vi "initialise.vi"(8 "error in (no error)":errorcluster, 11 "TrajectoryAN1106117SinglePoint in":refnum<class "TrajectoryAN1106117SinglePoint.lvclass">) -> (0 "error out":errorcluster, 3 "TrajectoryAN1106117SinglePoint out":refnum<class "TrajectoryAN1106117SinglePoint.lvclass">)   [LabVIEW 2010, in "TrajectoryAN1106117SinglePoint.lvclass"]
uses:
  TrajectoryAN1106117SinglePoint.lvclass
  TrajectoryDL091126GenericVoxel/TrajectoryDL091126GenericVoxel/TrajectoryDL091126GenericVoxel.lvclass
  common/enumerations/x_y_z_enumeration.ctl
  common/enumerations/functional_global_action_enum.ctl
  TrajectoryAN1106117SinglePoint.lvclass/TrajectoryAN1106117SinglePoint.ctl
  common/classes/ImageCollection/ImageCollection/ImageCollection.lvclass
  common/classes/Image/Image/Image.lvclass
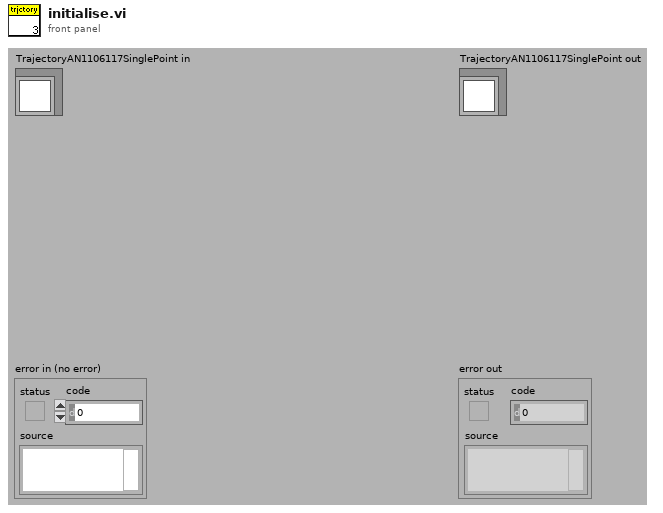
[diagram p1: front panel]
types:
  T1 = typedef "functional_global_action_enum.ctl" = enum16{"get", "set", "reset"}
  T2 = typedef "x_y_z_enumeration.ctl" = enum16{"x", "y", "z"}
  T3 = cluster{"Global Rectangle":dbl[unit][], "Contours":cluster{"Contour Type":u32, "ROI Type":u32, "Points":dbl[unit][]}[]}[]
  T4 = cluster{"Global Rectangle":dbl[unit][], "Contours":cluster{"Contour Type":u32, "ROI Type":u32, "Points":dbl[unit][]}[]}
  T5 = cluster{"Contour Type":u32, "ROI Type":u32, "Points":dbl[unit][]}[]
  T6 = cluster{"Contour Type":u32, "ROI Type":u32, "Points":dbl[unit][]}
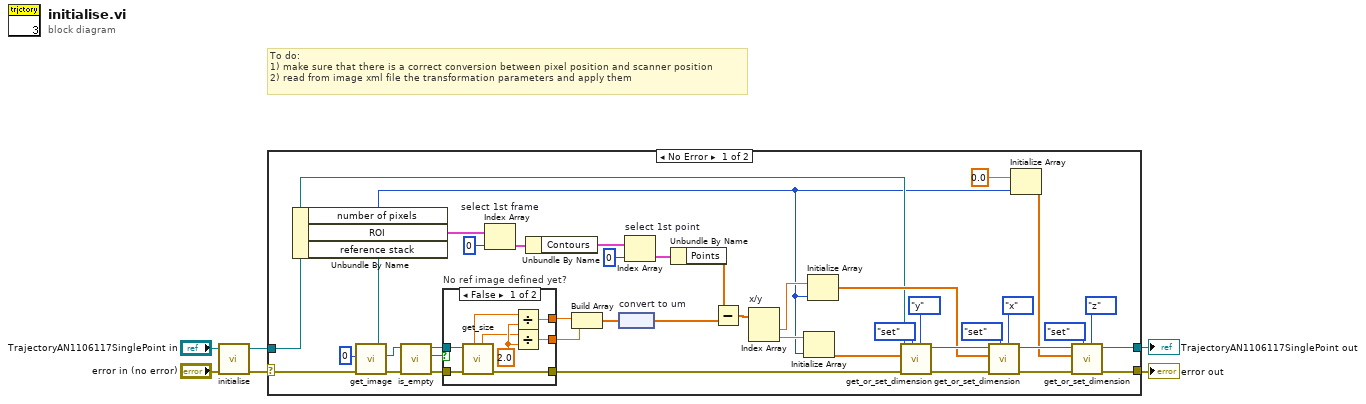
[diagram p0: block diagram]
diagram:
  # "To do:\n1) make sure that there is a correct conversion between pixel position and scanner position\n2) read from image xml file the transformation parameters and apply them"
  n1 = call-parent "initialise.vi"("error in (no error)"="error in (no error)", "GenericTrajectory in"="TrajectoryAN1106117SinglePoint in") -> ("error out"=w6:errorcluster, "GenericTrajectory out"=w5:refnum<class "TrajectoryAN1106117SinglePoint.lvclass">)  [unwired: 8 in]
  n2 = case shown="No Error" w6 {
    selector: w6 -> [w19 w58]
    tunnel: [w30 w58] -> w1
    tunnel: w5 -> [w25 w57]
    tunnel: [w29 w57] -> w2
    frame No Error {
      n3 = Unbundle By Name(w25) -> ("number of pixels"=w7:i32, "ROI"=w47:T3, "reference stack"=w20:refnum<class "ImageCollection.lvclass">)
      n4 = call-dynamic "get_image.vi"("error in (no error)"=w19, "index"=0, "ImageCollection in"=w20) -> ("error out"=w22:errorcluster, "Image.lvclass"=w21:refnum<class "Image.lvclass">)  [unwired: 6 in, 1 out]
      n5 = call-dynamic "is_empty.vi"("error in (no error)"=w22, "Image in"=w21) -> ("error out"=w23:errorcluster, "emtpy?"=w17:bool, "Image out"=w18:refnum<class "Image.lvclass">)  [unwired: 7 in]
      n6 = case "No ref image defined yet?" shown="False" w17 {
        tunnel: [w55 w56] -> w8
        tunnel: [w52 _] -> w16
        tunnel: [w50 _] -> w15
        tunnel: w23 -> [w49 w56]
        tunnel: w18 -> [w48 _]
        frame False {
          w54 = 2.0 ("y")
          n7 = call-dynamic "get_size.vi"("error in (no error)"=w49, "Image in"=w48) -> ("error out"=w55:errorcluster, "physical size y"=w51:dbl, "physical size x"=w53:dbl)  [unwired: 2 in, 5 out]
          n8 = Divide(x=w53, y=w54) -> (x/y=w52:dbl)
          n9 = Divide(x=w51, y=w54) -> (x/y=w50:dbl)
        }
        frame True {
        }
      }
      n10 = Index Array "select 1st frame"(array=w47, index=0) -> (element=w45:T4)
      n11 = Unbundle By Name(w45) -> ("Contours"=w43:T5)
      n12 = Build Array(w16, w15) -> (w14:dbl[])
      n13 = node "convert to um"(w14) -> (w13:dbl[unit][])
      n14 = Index Array "select 1st point"(array=w43, index=0) -> (element=w42:T6)
      n15 = Unbundle By Name(w42) -> ("Points"=w12:dbl[unit][])
      n16 = Subtract(x=w12, y=w13) -> (x-y=w11:dbl[unit][])
      n17 = Index Array "x/y"(array=w11) -> (element #1=w10:dbl[unit], element #2=w9:dbl[unit])  [unwired: 2 in]
      n18 = Initialize Array(w9, w7) -> (w35:dbl[unit][])
      n19 = Initialize Array(w10, w7) -> (w34:dbl[unit][])
      n20 = call-dynamic "get_or_set_dimension.vi"("dimension"=x_y_z_enumeration."y", "action"=functional_global_action_enum."set", "error in (no error)"=w8, "pixel values in (single dimension)"=w35, "GenericTrajectory in"=w25) -> ("error out"=w37:errorcluster, "GenericTrajectory out"=w36:refnum<class "TrajectoryAN1106117SinglePoint.lvclass">)  [unwired: 4 in, 1 out]
      n21 = call-dynamic "get_or_set_dimension.vi"("dimension"=x_y_z_enumeration."x", "action"=functional_global_action_enum."set", "error in (no error)"=w37, "pixel values in (single dimension)"=w34, "GenericTrajectory in"=w36) -> ("error out"=w31:errorcluster, "GenericTrajectory out"=w28:refnum<class "TrajectoryAN1106117SinglePoint.lvclass">)  [unwired: 4 in, 1 out]
      n22 = Initialize Array(dbl[unit] 0.0 ("element"), w7) -> (w26:dbl[unit][])
      n23 = call-dynamic "get_or_set_dimension.vi"("dimension"=x_y_z_enumeration."z", "action"=functional_global_action_enum."set", "error in (no error)"=w31, "pixel values in (single dimension)"=w26, "GenericTrajectory in"=w28) -> ("error out"=w30:errorcluster, "GenericTrajectory out"=w29:refnum<class "TrajectoryAN1106117SinglePoint.lvclass">)  [unwired: 4 in, 1 out]
    }
    frame Error {
    }
  }
  "error out" <- w1
  "TrajectoryAN1106117SinglePoint out" <- w2
